vi "参数设置.vi"(0 "X轴速度":dbl, 1 "精度":dbl, 2 "细分设置":dbl, 3 "等待时间":dbl, 5 "X轴回零速度":dbl, 9 "Y轴速度":dbl, 11 "Y轴回零速度":dbl) -> (4 "X轴速度":dbl, 6 "X轴回零速度":dbl, 10 "Y轴速度":dbl, 12 "精度":dbl, 13 "细分设置":dbl, 14 "等待时间":dbl, 15 "Y轴回零速度":dbl)   [LabVIEW 2016]
panel:
  in  "确定":bool
  in  "选项卡控件":enum32{"控制参数", "X轴", "Y轴"}(tab)
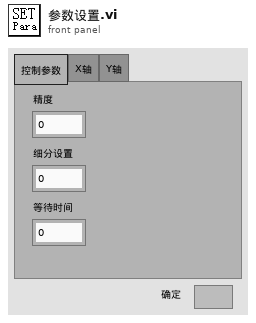
[diagram p1: front panel]
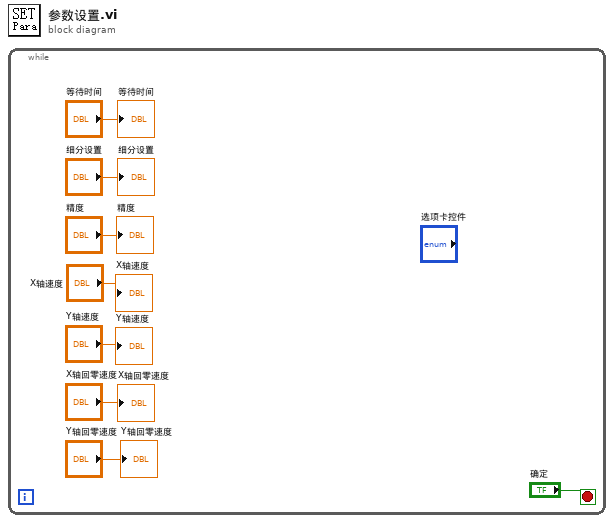
[diagram p0: block diagram]
diagram:
  n1 = while {
    stop <- "确定" stop-if-true
    "等待时间" <- "等待时间"
    "细分设置" <- "细分设置"
    "精度" <- "精度"
    "X轴速度" <- "X轴速度"
    "Y轴速度" <- "Y轴速度"
    "X轴回零速度" <- "X轴回零速度"
    "Y轴回零速度" <- "Y轴回零速度"
  }
